vi "Integer Mean.vi"(11 "Integer Array":u8[](array[numeric])) -> (3 "Numeric":i64)   [LabVIEW 2014]
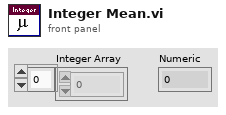
[diagram p1: front panel]
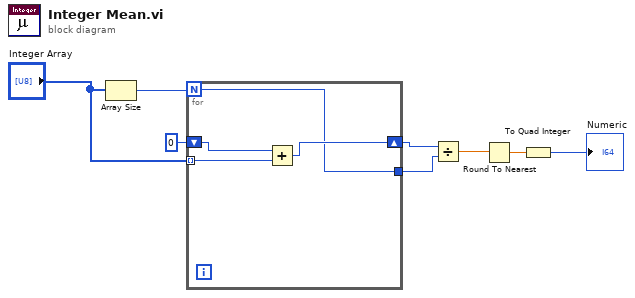
[diagram p0: block diagram]
diagram:
  n1 = Array Size(array="Integer Array") -> (size(s)=w5:i32)
  n2 = for {
    N: w5 -> [w9]
    shift-right: [w10] -> w6
    shift-left: u8 0 -> [w12]
    tunnel: "Integer Array" -> [w11] mode=indexing
    tunnel: [w9] -> w7
    n3 = Add(x=w12, y=w11) -> (x+y=w10:u8)
  }
  n4 = Divide(x=w6, y=w7) -> (x/y=w4:dbl)
  n5 = Round To Nearest(number=w4) -> (nearest integer value=w3:dbl)
  n6 = To Quad Integer(1:w3) -> (0:→"Numeric":i64)
